vi "Do.vi"(8 "error in (no error)":errorcluster, 10 "Actor in":refnum<class "Actor.lvclass">, 11 "Register PVs Msg in":refnum<class "Register PVs Msg.lvclass">) -> (0 "error out":errorcluster, 2 "Actor out":refnum<class "Actor.lvclass">)   [LabVIEW 2014, in "CS++ControllerActor.lvlib" / "Register PVs Msg.lvclass"]
doc: "(<B>Filename</B>: Actor Framework.lvlib:Message.lvclass:Do.vi)\n\nDefines what a message does when it is received by an actor. Generally, a message instructs an actor to invoke one of its methods. By default, this method does nothing. A child class must override it to define behavior. Create a child class by using the Actor Framework Message Maker dialog box."
uses:
  Register PVs Msg.lvclass
  <vilib>/ActorFramework/Actor/Actor.lvclass
  CS++ControllerActor/CS++ControllerActor.lvclass
  CS++PVMonitor Messages/CS++PVUpdate Msg/CS++PVUpdate Msg.lvclass/CS++PVUpdate Msg.ctl
  Classes/CS++ProcessVariables/ProcessVariable/PV.lvclass/PV.ctl
  Register PVs Msg.lvclass/Register PVs Msg.ctl
  Classes/CS++ProcessVariables/ProcessVariable/PV.lvclass
  CS++PVMonitor Messages/CS++PVUpdate Msg/CS++PVUpdate Msg.lvclass
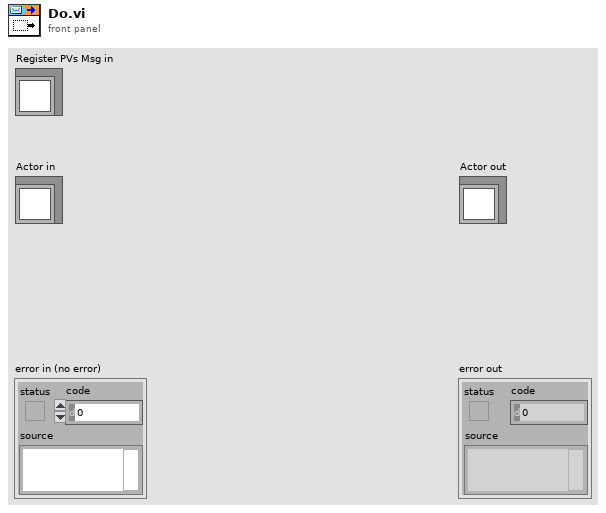
[diagram p1: front panel]
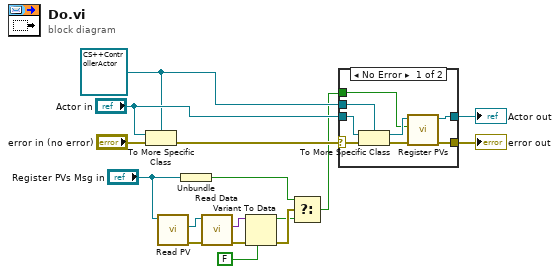
[diagram p0: block diagram]
diagram:
  w11 = refnum<class "CS++ControllerActor.lvclass"> refnum ("Actor Type")
  n1 = To More Specific Class(target class=w11, reference="Actor in", error in="error in (no error)") -> (error out=w15:errorcluster)  [unwired: 1 out]
  n2 = call "Read PV.vi"("CS++PVUpdate Msg in"="Register PVs Msg in") -> ("error out"=w10:errorcluster, "PV"=w9:refnum<class "PV.lvclass">)  [unwired: 8 in, 1 out]
  n3 = Unbundle("Register PVs Msg in") -> (w2:bool)
  n4 = call "Read Data.vi"("error in (no error)"=w10, "PV in"=w9) -> ("error out"=w6:errorcluster, "Data"=w7:variant)  [unwired: 7 in, 1 out]
  n5 = Variant To Data(error in=w6, type=FALSE, Variant=w7) -> (data=w3:bool, error out=w4:errorcluster)
  n6 = Select(t=w2, s=w4, f=w3) -> (s? t:f=w1:bool)
  n7 = case shown="No Error" w15 {
    selector: w15 -> [w24 w26]
    tunnel: [w19 w26] -> w14
    tunnel: [w18 w25] -> w13
    tunnel: "Actor in" -> [w23 w25]
    tunnel: w11 -> [w22 _]
    tunnel: w1 -> [w17 _]
    frame No Error {
      n8 = To More Specific Class ("Actor Cast")(target class=w22, reference=w23, error in=w24) -> (specific class reference=w21:refnum<class "CS++ControllerActor.lvclass">, error out=w20:errorcluster)
      n9 = call "Register PVs.vi"("error in (no error)"=w20, "Activate?"=w17, "CS++ControllerActor in"=w21) -> ("error out"=w19:errorcluster, "CS++ControllerActor out"=w18:refnum<class "CS++ControllerActor.lvclass">)  [unwired: 7 in]
    }
    frame Error {
    }
  }
  "error out" <- w14
  "Actor out" <- w13
